vi "Modbus_采集温度数据.vi"(8 "error in (no error)":errorcluster caption="错误输入（无错误）", 11 "Mod":T1) -> (0 "error out":errorcluster caption="错误输出", 3 "Mod 2":T1)   [LabVIEW 2018]
uses:
  <vilib>/Modbus/master/Modbus Master.lvclass
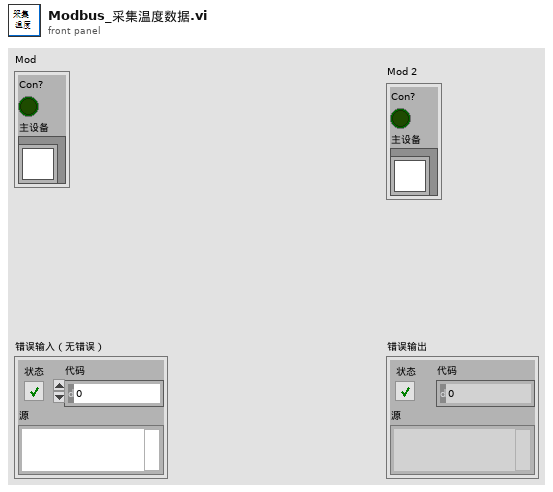
[diagram p1: front panel]
types:
  T1 = cluster{"Con?":bool, "主设备":refnum<class "Modbus Master.lvclass">}
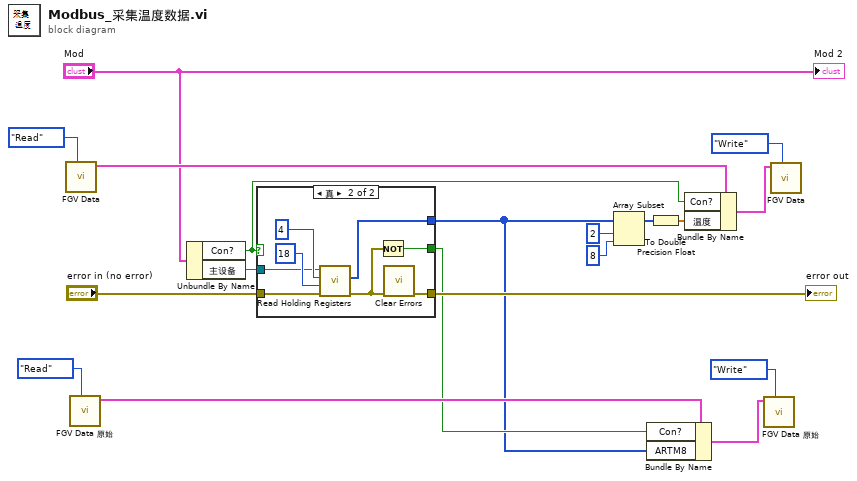
[diagram p0: block diagram]
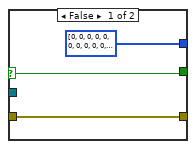
[diagram p2: hidden frame]
diagram:
  n1 = call "FGV Data.vi"("Action"=enum16{"Initial", "Read", "Write"}."Read") -> ("Data OUT"=w15:cluster{"Con?":bool, "温度":dbl[]})  [unwired: 9 in, 1 out]
  n2 = call "FGV Data 原始.vi"("Action"=enum16{"Initial", "Read", "Write"}."Read") -> ("Data OUT"=w5:cluster{"Con?":bool, "ARTM8":u16[]})  [unwired: 9 in, 1 out]
  n3 = Unbundle By Name("Mod") -> ("Con?"=w1:bool, "主设备"=w18:refnum<class "Modbus Master.lvclass">)
  n4 = case shown="真" w1 {
    selector: w1 -> [w20 _]
    tunnel: "error in (no error)" -> [w22 w30]
    tunnel: w18 -> [_ w27]
    tunnel: [w22 w24] -> w12
    tunnel: [u16[] [0, 0, 0, 0, 0, 0, 0, 0, 0, 0, 0, 0, 0, 0, 0, 0, 0, 0] ("register values") w26] -> w2
    tunnel: [w20 w23] -> w3
    frame False {
    }
    frame True {
      n5 = call-dynamic "Read Holding Registers.vi"("error in (no error)"=w30, "number of holding registers"=u16 18, "starting address"=u16 4, "Modbus master in"=w27) -> ("error out"=w25:errorcluster, "register values"=w26:u16[])  [unwired: 5 in, 1 out]
      n6 = Not(x=w25) -> (.not. x?=w23:bool)
      n7 = call <vilib>:"Clear Errors.vi"("error in (no error)"=w25) -> ("error out"=w24:errorcluster)  [unwired: 5 in, 1 out]
    }
  }
  "error out" <- w12
  n8 = Array Subset(array=w2, index=2 ("索引"), length=8 ("长度")) -> (w11:u16[])
  n9 = Bundle By Name(cluster=w5, "Con?"=w3, "ARTM8"=w2) -> (w4:cluster{"Con?":bool, "ARTM8":u16[]})
  n10 = To Double Precision Float(number=w11) -> (double precision float=w14:dbl[])
  n11 = Bundle By Name(cluster=w15, "Con?"=w1, "温度"=w14) -> (w13:cluster{"Con?":bool, "温度":dbl[]})
  n12 = call "FGV Data 原始.vi"("Action"=enum16{"Initial", "Read", "Write"}."Write", "Data IN"=w4) -> ()  [unwired: 8 in, 2 out]
  n13 = call "FGV Data.vi"("Action"=enum16{"Initial", "Read", "Write"}."Write", "Data IN"=w13) -> ()  [unwired: 8 in, 2 out]
  "Mod 2" <- "Mod"
